vi "I8.vi"(1 "Numeric Input":i8) -> (0 "Numeric Output":i8)   [LabVIEW 2011]
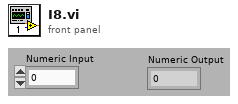
[diagram p1: front panel]
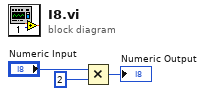
[diagram p0: block diagram]
diagram:
  n1 = Multiply(x="Numeric Input", y=i8 2) -> (x*y=→"Numeric Output":i8)
